vi "Build.vi"(9 "XYZTheta":dbl[](array[numeric]), 10 "Pattern Coordinates":dbl[][](array[numeric]), 11 "CAD Dispense in":refnum<class "CAD Dispense.lvclass">) -> (1 "Starting Coordinates":dbl[](array[numeric]), 3 "CAD Dispense out":refnum<class "CAD Dispense.lvclass">)   [LabVIEW 2016, in "CAD Dispense.lvclass"]
uses:
  CAD Dispense.lvclass
  CAD Dispense.lvclass/CAD Dispense.ctl
  <vilib>/Analysis/coordinate.llb/2D Cartesian Coordinate Rotation (Scalar).vi
  <vilib>/Analysis/NI_AALPro.lvlib
panel:
  out "array w/ subset deleted 2":T1(array[cluster])
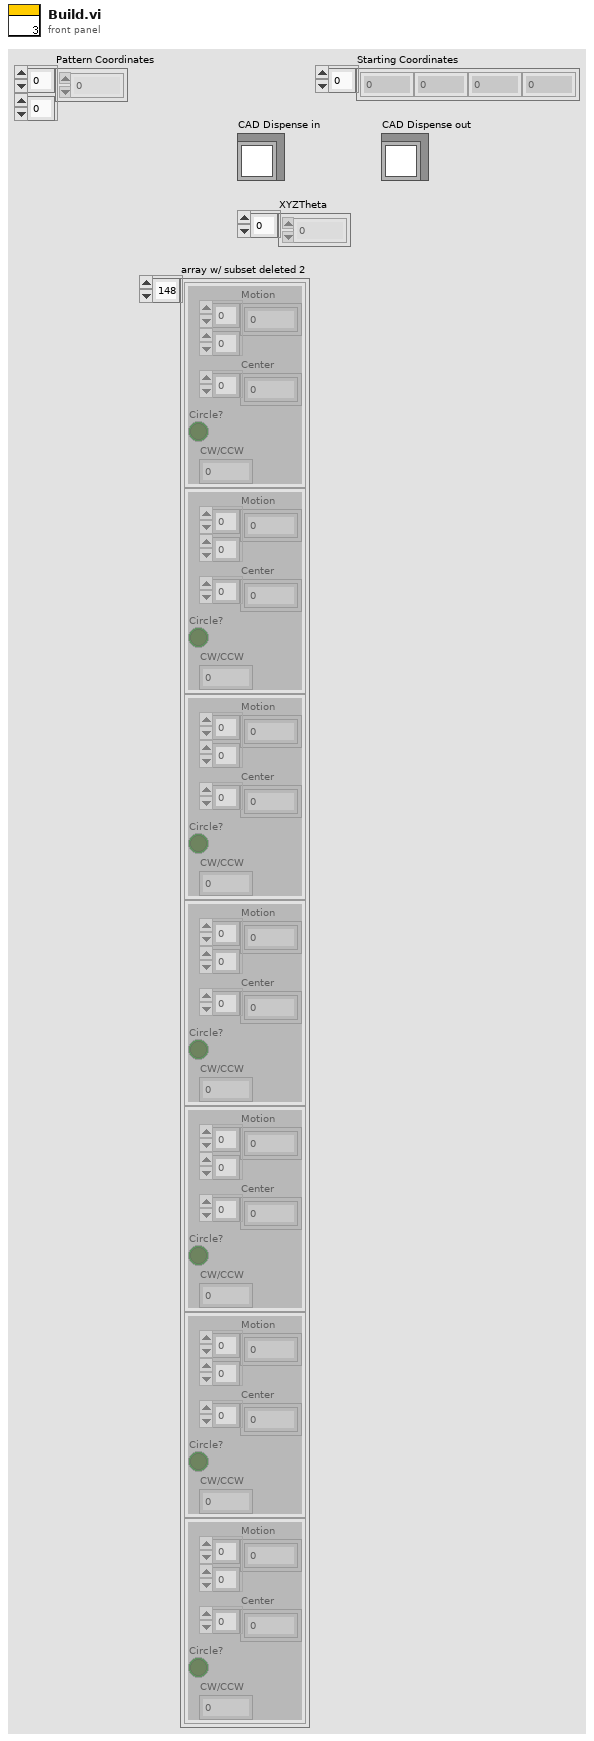
[diagram p1: front panel]
types:
  T1 = cluster{"Motion":dbl[][], "Center":dbl[], "Circle?":bool, "CW/CCW":dbl}[]
  T2 = cluster{"Motion":dbl[][], "Center":dbl[], "Circle?":bool, "CW/CCW":dbl}
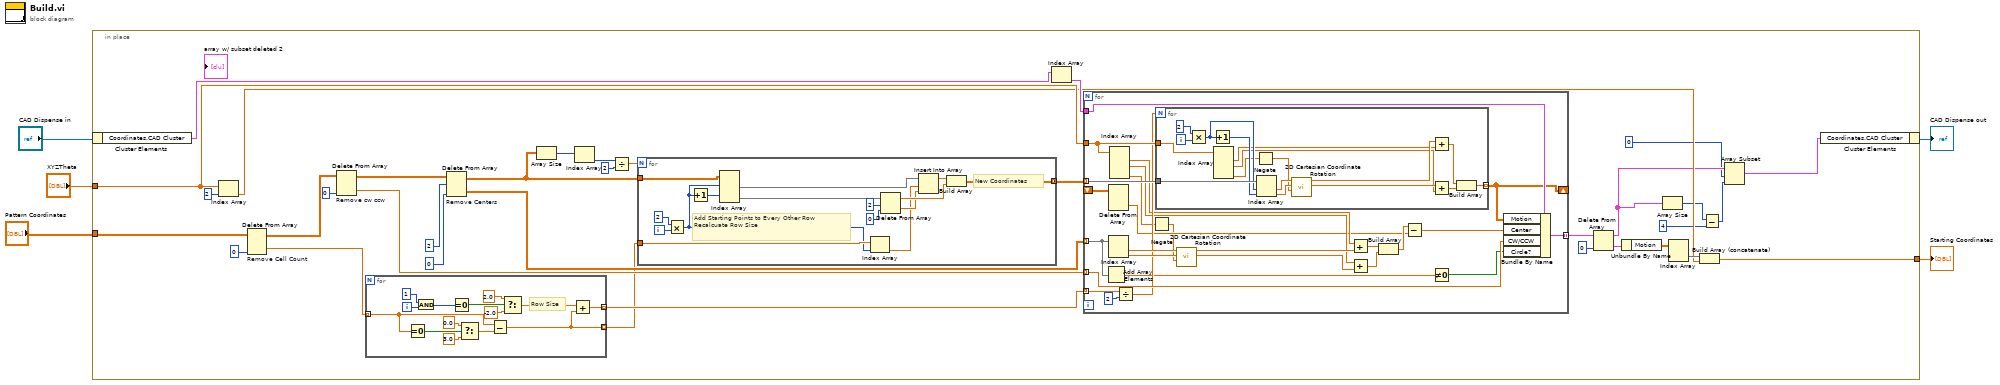
[diagram p0: block diagram]
diagram:
  n1 = in-place {
    in-place-border: "XYZTheta" -> [w15]
    in-place-border: "Pattern Coordinates" -> [w27]
    in-place-border: [w12] -> w3
    n2 = in-place-cluster #1("CAD Dispense in") -> ("Coordinates.CAD Cluster"=w29:T1)
    n3 = Index Array(array=w15, index=2) -> (element=w13:dbl)
    n4 = Delete From Array "Remove Cell Count"(array=w27, index (col)=0 ("disabled index (col)")) -> (deleted portion=w23:dbl[], array with subset deleted=w34:dbl[][])  [unwired: 2 in]
    n5 = Delete From Array "Remove cw ccw"(array=w34, index (col)=0 ("disabled index (col)")) -> (deleted portion=w39:dbl[], array with subset deleted=w35:dbl[][])  [unwired: 2 in]
    n6 = for {
      tunnel: w23 -> [w50] mode=indexing
      tunnel: [w42] -> w22 mode=indexing
      tunnel: [w41] -> w21 mode=indexing
      i -> [w43]
      # "Row Size"
      n7 = Equal To 0?(x=w50) -> (x = 0?=w51:bool)
      n8 = And(x=1, y=w43) -> (x .and. y?=w46:i32)
      n9 = Equal To 0?(x=w46) -> (x = 0?=w44:bool)
      n10 = Select(t=0.0, s=w51, f=3.0) -> (s? t:f=w54:dbl)
      n11 = Subtract(x=w50, y=w54) -> (x-y=w41:dbl)
      n12 = Select(t=2.0, s=w44, f=-2.0) -> (s? t:f=w47:dbl)
      n13 = Add(x=w47, y=w41) -> (x+y=w42:dbl)
    }
    n14 = Delete From Array "Remove Centers"(array=w35, length=2, index (col)=0 ("disabled index (col)")) -> (deleted portion=w40:dbl[][], array with subset deleted=w36:dbl[][])  [unwired: 1 in]
    n15 = Array Size(array=w36) -> (size(s)=w37:i32[])
    n16 = Index Array(array=w37) -> (element=w26:i32)  [unwired: 1 in]
    n17 = Divide(x=w26, y=2) -> (x/y=w24:dbl)
    n18 = for {
      N: w24 -> [_]
      tunnel: w36 -> [w112]
      tunnel: [w104] -> w38 mode=concatenating
      tunnel: w21 -> [w99]
      i -> [w105]
      # "New Coordinates"
      # "Add Starting Points to Every Other Row\nRecalcuate Row Size"
      n19 = Multiply(x=2, y=w105) -> (x*y=w98:i32)
      n20 = Increment(x=w98) -> (x+1=w100:i32)
      n21 = Index Array(array=w112, index (row) #1=w98, index (row) #2=w100) -> (element #1=w108:dbl[], element #2=w110:dbl[])  [unwired: 2 in]
      n22 = Index Array(array=w99, index=w98) -> (element=w101:dbl)
      n23 = Delete From Array(array=w110, length=2, index=0) -> (deleted portion=w102:dbl[], array with subset deleted=w106:dbl[])
      n24 = Insert Into Array(array=w108, index=w101, new element=w102) -> (w107:dbl[])
      n25 = Build Array(w107, w106) -> (w104:dbl[][])
    }
    n26 = Index Array(array=w29) -> (element=w28:T2)  [unwired: 1 in]
    n27 = for {
      tunnel: w22 -> [w78] mode=indexing
      tunnel: w38 -> [w73] mode=indexing
      tunnel: w39 -> [w76] mode=indexing
      tunnel: w40 -> [w72] mode=indexing
      tunnel: w15 -> [w79]
      tunnel: w28 -> [w77]
      tunnel: [w74] -> w18 mode=indexing
      shift-right: [w62] -> _
      shift-left: _ -> [w60]
      n28 = Add Array Elements(numeric array=w72) -> (sum=w57:dbl)
      n29 = Delete From Array(array=w60) -> (deleted portion=w59:dbl[])  [unwired: 3 in, 1 out]
      n30 = Index Array(array=w72) -> (element #1=w71:dbl, element #2=w70:dbl)  [unwired: 2 in]
      n31 = Index Array(array=w79) -> (element #1=w68:dbl, element #2=w63:dbl, element #4=w56:dbl)  [unwired: 4 in, 1 out]
      n32 = Divide(x=w78, y=2) -> (x/y=w69:dbl)
      n33 = Negate(x=w56) -> (-x=w55:dbl)
      n34 = for {
        N: w69 -> [_]
        tunnel: w73 -> [w97]
        tunnel: [w83] -> w62 mode=indexing
        tunnel: w79 -> [w93]
        i -> [w84]
        n35 = Multiply(x=2, y=w84) -> (x*y=w95:i32)
        n36 = Increment(x=w95) -> (x+1=w94:i32)
        n37 = Index Array(array=w93) -> (element #1=w86:dbl, element #2=w85:dbl, element #4=w82:dbl)  [unwired: 4 in, 1 out]
        n38 = Negate(x=w82) -> (-x=w81:dbl)
        n39 = Index Array(array=w97, index #1=w95, index #2=w94) -> (element #1=w89:dbl, element #2=w88:dbl)
        n40 = call-poly <vilib>:"2D Cartesian Coordinate Rotation.vi"("theta"=w81, "y"=w88, "x"=w89) -> ("y out"=w92:dbl, "x out"=w87:dbl)  [unwired: 6 in, 1 out]
        n41 = Add(x=w87, y=w86) -> (x+y=w91:dbl)
        n42 = Add(x=w92, y=w85) -> (x+y=w90:dbl)
        n43 = Build Array(w91, w90) -> (w83:dbl[])
      }
      n44 = call-poly <vilib>:"2D Cartesian Coordinate Rotation.vi"("theta"=w55, "y"=w70, "x"=w71) -> ("y out"=w65:dbl, "x out"=w67:dbl)  [unwired: 6 in, 1 out]
      n45 = Add(x=w68, y=w67) -> (x+y=w66:dbl)
      n46 = Add(x=w63, y=w65) -> (x+y=w64:dbl)
      n47 = Build Array(w66, w64) -> (w61:dbl[])
      n48 = Subtract(x=w61, y=w59) -> (x-y=w58:dbl[])
      n49 = Not Equal To 0?(x=w57) -> (x != 0?=w75:bool)
      n50 = Bundle By Name(cluster=w77, "Motion"=w62, "Center"=w58, "CW/CCW"=w76, "Circle?"=w75) -> (w74:T2)
    }
    n51 = Delete From Array(array=w18, index=0) -> (deleted portion=w20:T2, array with subset deleted=w11:T1)  [unwired: 1 in]
    n52 = Unbundle By Name(w20) -> ("Motion"=w17:dbl[][])
    n53 = Array Size(array=w11) -> (size(s)=w9:i32)
    n54 = Index Array(array=w17) -> (element=w16:dbl[])  [unwired: 2 in]
    n55 = Build Array (concatenate)(w16, w13) -> (w12:dbl[])
    n56 = Subtract(x=w9, y=4) -> (x-y=w7:i32)
    n57 = Array Subset(array=w11, index=0, length=w7) -> (w6:T1)
    n58 = in-place-cluster #1("Coordinates.CAD Cluster"=w6) -> (→"CAD Dispense out":refnum<class "CAD Dispense.lvclass">)
  }
  "Starting Coordinates" <- w3
